vi "apply new date info.vi"(8 "error in":errorcluster, 11 "Cluster in":T1={"Running VI"=refnum, "Test VI"=refnum, "Q Ref"=refnum, "UE"=refnum, "Data"=variant, "Timeout"=-1, "ListBox[]"=[], "Source Path"=path "", "Delta Time"=0.0, "ExifInfo[]"=[], "ListIndex"=0, "counter"=0, "Format"=enum."Files Only", "total"=0, "Operation"=enum."Read Info", "Status"=""} {"ExifInfo[]"."New DateTime" format="%<%.3X>T"; "ExifInfo[]"."DateTimeOrginal" format="%<%.3X>T"}) -> (0 "error out":errorcluster, 3 "Cluster out":T1={"Running VI"=refnum, "Test VI"=refnum, "Q Ref"=refnum, "UE"=refnum, "Data"=variant, "Timeout"=-1, "ListBox[]"=[], "Source Path"=path "", "Delta Time"=0.0, "ExifInfo[]"=[], "ListIndex"=0, "counter"=0, "Format"=enum."Files Only", "total"=0, "Operation"=enum."Read Info", "Status"=""} {"ExifInfo[]"."New DateTime" format="%<%.3X>T"; "ExifInfo[]"."DateTimeOrginal" format="%<%.3X>T"})   [LabVIEW 2023, in "EXIF Modifier.lvlib"]
uses:
  EXIF Modifier.lvlib
  Controls/exif_consumer cluster.ctl
  Controls/exif_info cluster.ctl
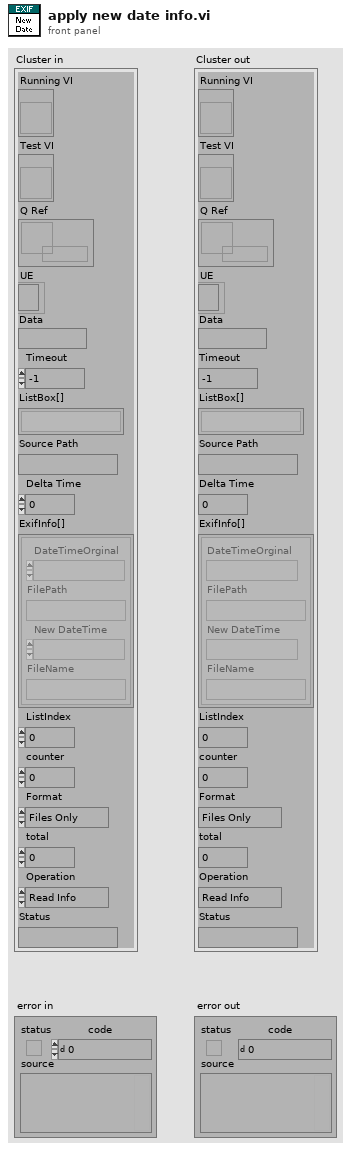
[diagram p1: front panel]
types:
  T1 = typedef "EXIF Modifier.lvlib/exif_consumer cluster.ctl" = cluster{"Running VI":refnum<vi>, "Test VI":refnum<vi>, "Q Ref":refnum<queue>, "UE":refnum<event-registration>, "Data":variant, "Timeout":i32, "ListBox[]":string[][], "Source Path":path, "Delta Time":dbl, "ExifInfo[]":T2[], "ListIndex":i32, "counter":i32, "Format":enum16{"Files Only", "Files Date", "All"}, "total":i32, "Operation":enum16{"Read Info", "Write Info"}, "Status":string}
  T2 = typedef "EXIF Modifier.lvlib/exif_info cluster.ctl" = cluster{"DateTimeOrginal":timestamp, "FilePath":path, "New DateTime":timestamp, "FileName":string}
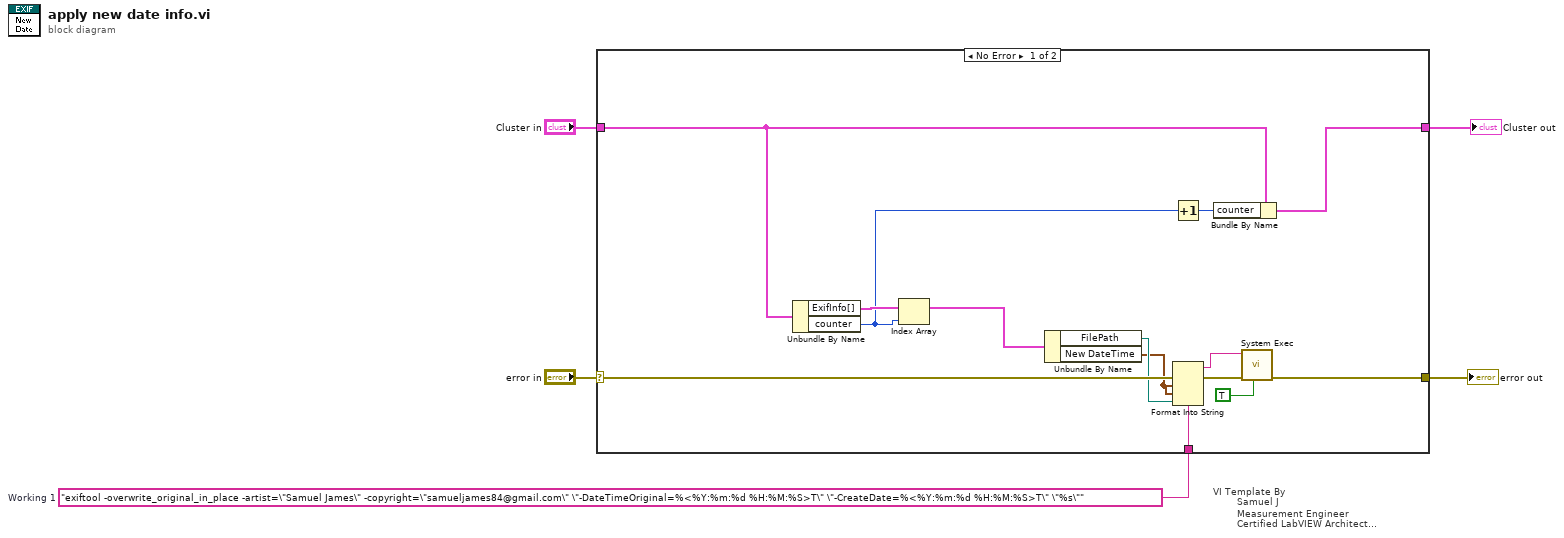
[diagram p0: block diagram]
diagram:
  w1 = "exiftool -overwrite_original_in_place -artist=\"Samuel James\" -copyright=\"samueljames84@gmail.com\" \"-DateTimeOriginal=%<%Y:%m:%d %H:%M:%S>T\" \"-CreateDate=%<%Y:%m:%d %H:%M:%S>T\" \"%s\""  # Working 1
  n1 = case "VI Template By\n        Samuel J\n        Measurement Engineer\n        Certified LabVIEW Architect\n        Vestas Technology R&D Chennai" shown="No Error" "error in" {
    selector: "error in" -> [w9 w21]
    tunnel: [w10 w21] -> w4
    tunnel: [w16 w20] -> w2
    tunnel: "Cluster in" -> [w17 w20]
    tunnel: w1 -> [w8 _]
    frame No Error {
      n2 = Unbundle By Name(w17) -> ("ExifInfo[]"=w19:T2[], "counter"=w15:i32)
      n3 = Index Array(array=w19, index=w15) -> (element=w18:T2)
      n4 = Unbundle By Name(w18) -> ("FilePath"=w7:path, "New DateTime"=w6:timestamp)
      n5 = Increment(x=w15) -> (x+1=w14:i32)
      n6 = Format Into String(format string=w8, error in=w9, w6, w6, w7) -> (resulting string=w12:string, error out=w13:errorcluster)  [unwired: 1 in]
      n7 = Bundle By Name(cluster=w17, "counter"=w14) -> (w16:T1)
      n8 = call <vilib>:"System Exec.vi"("run minimized? (F)"=TRUE, "error in (no error)"=w13, "command line"=w12) -> ("error out"=w10:errorcluster)  [unwired: 5 in, 3 out]
    }
    frame Error {
    }
  }
  "error out" <- w4
  "Cluster out" <- w2
